vi "Handle Multicolumn Listbox Settings.vi"(6 "Table Setting Name in":string, 7 "Write? (F:Read)":bool, 8 "error in (no error)":errorcluster, 9 "Table Ref":refnum<vi>, 11 "Save Restore Settings in":refnum<class "Save Restore Settings.lvclass">) -> (0 "error out":errorcluster, 1 "Sub Controls":T1[](array[typedef]), 3 "Save Restore Settings out":refnum<class "Save Restore Settings.lvclass">)   [LabVIEW 2020, in "Save Restore Settings.lvclass"]
uses:
  <userlib>/_MGI/Application Control/MGI Save Restore Settings/Save Restore Settings.lvclass
  <userlib>/_MGI/Application Control/MGI Save Restore Settings/Control Info.ctl
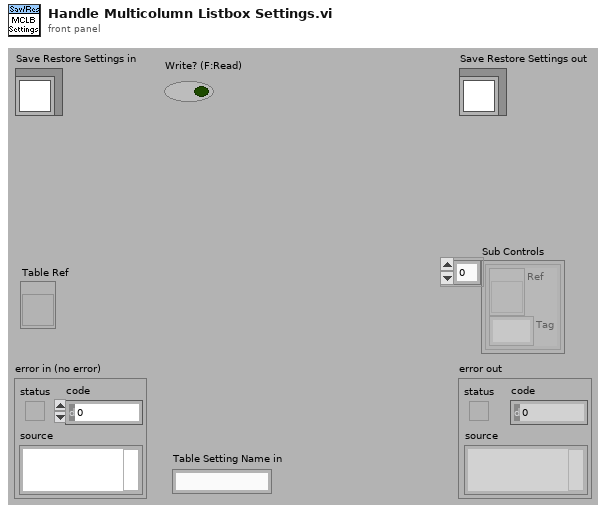
[diagram p1: front panel]
types:
  T1 = typedef "Save Restore Settings.lvclass/Control Info.ctl" = cluster{"Ref":refnum<vi>, "Tag":string}
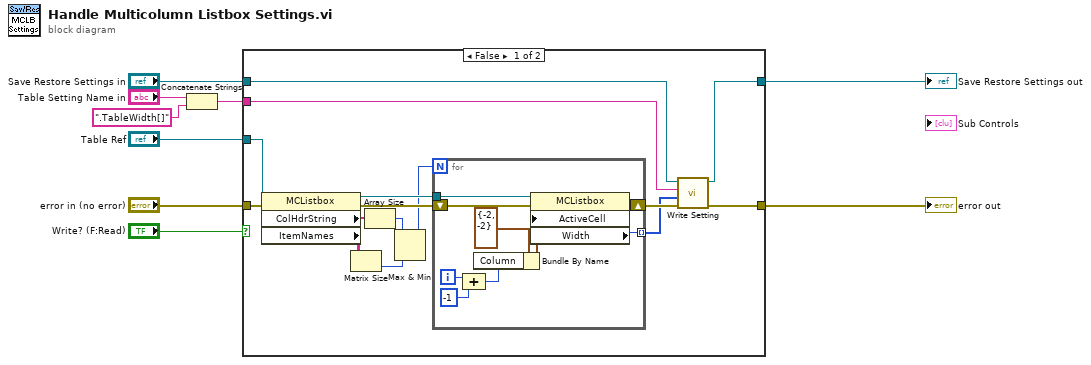
[diagram p0: block diagram]
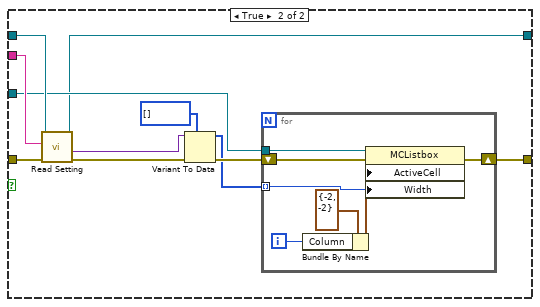
[diagram p2: hidden frame]
diagram:
  n1 = Concatenate Strings("Table Setting Name in", ".TableWidth[]" ("string")) -> (w2:string)
  n2 = case shown="False" "Write? (F:Read)" {
    tunnel: "Table Ref" -> [w17 w36]
    tunnel: "error in (no error)" -> [w18 w43]
    tunnel: "Save Restore Settings in" -> [w24 w41]
    tunnel: [w23 w34] -> w6
    tunnel: [w22 w40] -> w5
    tunnel: w2 -> [w21 w42]
    frame False {
      n3 = property class="MCListbox"(reference=w17, error in=w18) -> (reference out=w15:refnum<vi>, error out=w16:errorcluster, "ColHdrString"=w14:string[], "ItemNames"=w13:string[][])
      n4 = Matrix Size(0:w13) -> (2:w11:i32)  [unwired: 1 out]
      n5 = Array Size(array=w14) -> (size(s)=w12:i32)
      n6 = Max & Min(x=w12, y=w11) -> (max(x,y)=w10:i32)  [unwired: 1 out]
      n7 = for {
        N: w10 -> [_]
        shift-right: [w26] -> w20
        shift-left: w16 -> [w30]
        tunnel: w15 -> [w33]
        tunnel: [w25] -> w19 mode=indexing
        i -> [w29]
        n8 = Compound Arithmetic op=ADD(w29, -1 ("y")) -> (w28:i32)
        n9 = Bundle By Name(cluster=cluster{"Row":i32, "Column":i32} {"Row"=-2, "Column"=-2} ("Active Cell:Active Cell"), "Column"=w28) -> (w31:cluster{"Row":i32, "Column":i32})
        n10 = property class="MCListbox"(reference=w33, error in=w30, "ActiveCell"=w31) -> (error out=w26:errorcluster, "Width"=w25:u32)  [unwired: 1 out]
      }
      n11 = call-dynamic "Write Setting.vi"("error in (no error)"=w20, "Tag Attribute"=w19, "Tag Name"=w21, "Save Restore Settings in"=w24) -> ("error out"=w22:errorcluster, "Save Restore Settings out"=w23:refnum<class "Save Restore Settings.lvclass">)  [unwired: 6 in]
    }
    frame True {
      n12 = call-dynamic "Read Setting.vi"("error in (no error)"=w43, "Tag Name"=w42, "Save Restore Settings in"=w41) -> ("error out"=w44:errorcluster, "Tag Attribute"=w38:variant, "Save Restore Settings out"=w34:refnum<class "Save Restore Settings.lvclass">)  [unwired: 6 in]
      n13 = Variant To Data(error in=w44, type=u32[] [], Variant=w38) -> (data=w35:u32[], error out=w39:errorcluster)
      n14 = for {
        shift-right: [w50] -> w40
        shift-left: w39 -> [w45]
        tunnel: w36 -> [w51]
        tunnel: w35 -> [w49] mode=indexing
        i -> [w47]
        n15 = Bundle By Name(cluster=cluster{"Row":i32, "Column":i32} {"Row"=-2, "Column"=-2} ("Active Cell:Active Cell"), "Column"=w47) -> (w46:cluster{"Row":i32, "Column":i32})
        n16 = property class="MCListbox"(reference=w51, error in=w45, "ActiveCell"=w46, "Width"=w49) -> (error out=w50:errorcluster)  [unwired: 1 out]
      }
    }
  }
  "error out" <- w5
  "Save Restore Settings out" <- w6
